vi "SID_test_dump_player.vi"() -> ()   [LabVIEW 2018]
doc: "This VI illustrates how to generate and play sine, square, sawtooth and triangle waveforms. You can change the frequency and type of the waveform generated as it plays continuously."
uses:
  SID_voice_reg.ctl
  SID_filter_reg.ctl
  <vilib>/sound2/lvsound2.llb/Sampling Mode.ctl
  <vilib>/sound2/lvsound2.llb/Sound Data Format.ctl
  <vilib>/sound2/lvsound2.llb/Sound Output Set Volume (Single).vi
  <vilib>/sound2/lvsound2.llb/Sound Output Write (DBL Single).vi
panel:
  in  "Filter":T1 {"vol" format="%0.2f"; "res" format="%0.2f"; "freq" format="%0.2f"}
  in  "VC3":T2 {"Duty" format="%0.2f"; "ADSR"."R" format="%0.2f"; "ADSR"."S" format="%0.2f"; "ADSR"."D" format="%0.2f"; "ADSR"."A" format="%0.2f"; "freq" format="%0.2f"}
  in  "VC1":T2 {"Duty" format="%0.2f"; "ADSR"."R" format="%0.2f"; "ADSR"."S" format="%0.2f"; "ADSR"."D" format="%0.2f"; "ADSR"."A" format="%0.2f"; "freq" format="%0.2f"}
  in  "VC2":T2 {"Duty" format="%0.2f"; "ADSR"."R" format="%0.2f"; "ADSR"."S" format="%0.2f"; "ADSR"."D" format="%0.2f"; "ADSR"."A" format="%0.2f"; "freq" format="%0.2f"}
  out "VC3":dbl[](graph)
  out "VC2":dbl[](graph)
  out "VC1":dbl[](graph)
  out "data size(s)":i32
  out "time Audio":u32
  out "time SID":u32
  in  "Volume":dbl=0.5
  out "Wave":dbl[](graph)
  in  "Stop":bool
  in  "Device ID":u32
  # "D:\\work\\experimets\\C64\\a_mind_is_born_LV.wav"
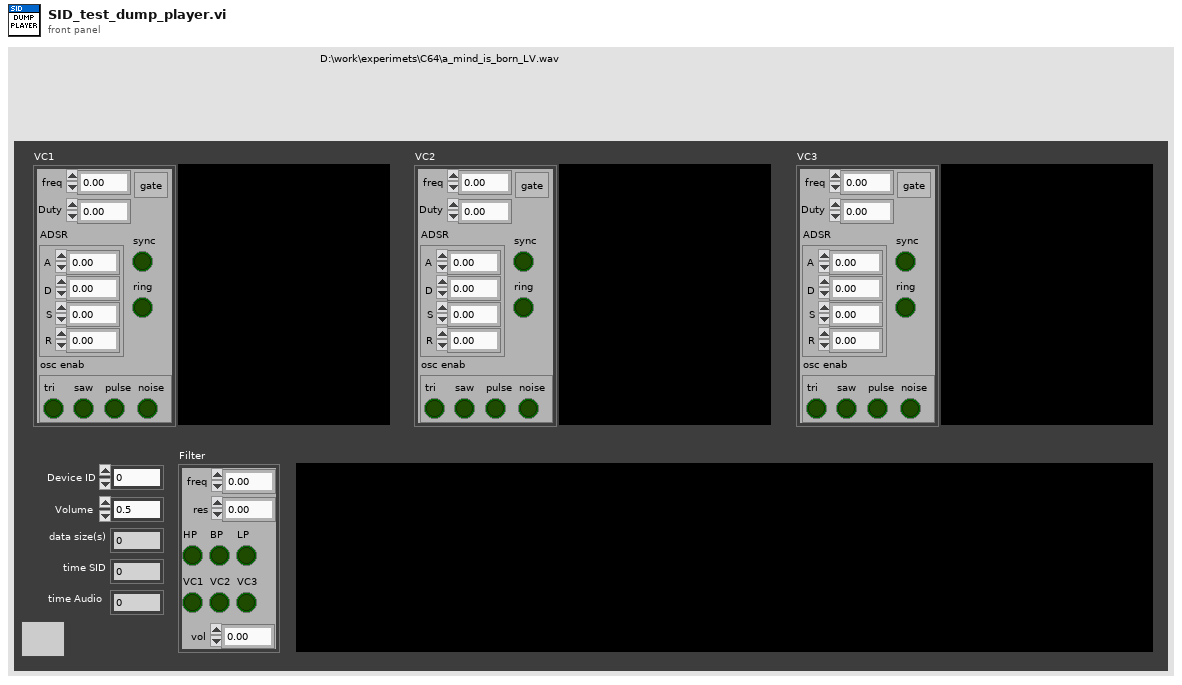
[diagram p1: front panel]
types:
  T1 = typedef "SID_filter_reg.ctl" = cluster{"freq":dbl, "res":dbl, "HP":bool, "BP":bool, "LP":bool, "VC1":bool, "VC2":bool, "VC3":bool, "vol":dbl}
  T2 = typedef "SID_voice_reg.ctl" = cluster{"freq":dbl, "gate":bool, "ADSR":cluster{"A":dbl, "D":dbl, "S":dbl, "R":dbl}, "Duty":dbl, "osc enab":cluster{"tri":bool, "saw":bool, "pulse":bool, "noise":bool}, "sync":bool, "ring":bool}
  T3 = enum16{"idle", "pre-attack", "attack", "pre-decay", "decay", "sustain", "pre-release", "release"}
  T4 = typedef "Sound Data Format.ctl" = cluster{"sample rate (S/s)":dbl, "number of channels":i32, "bits per sample":i32}
  T5 = typedef "Sampling Mode.ctl" = i32
  T6 = typedef "Sound Output Task ID.ctl" = u32
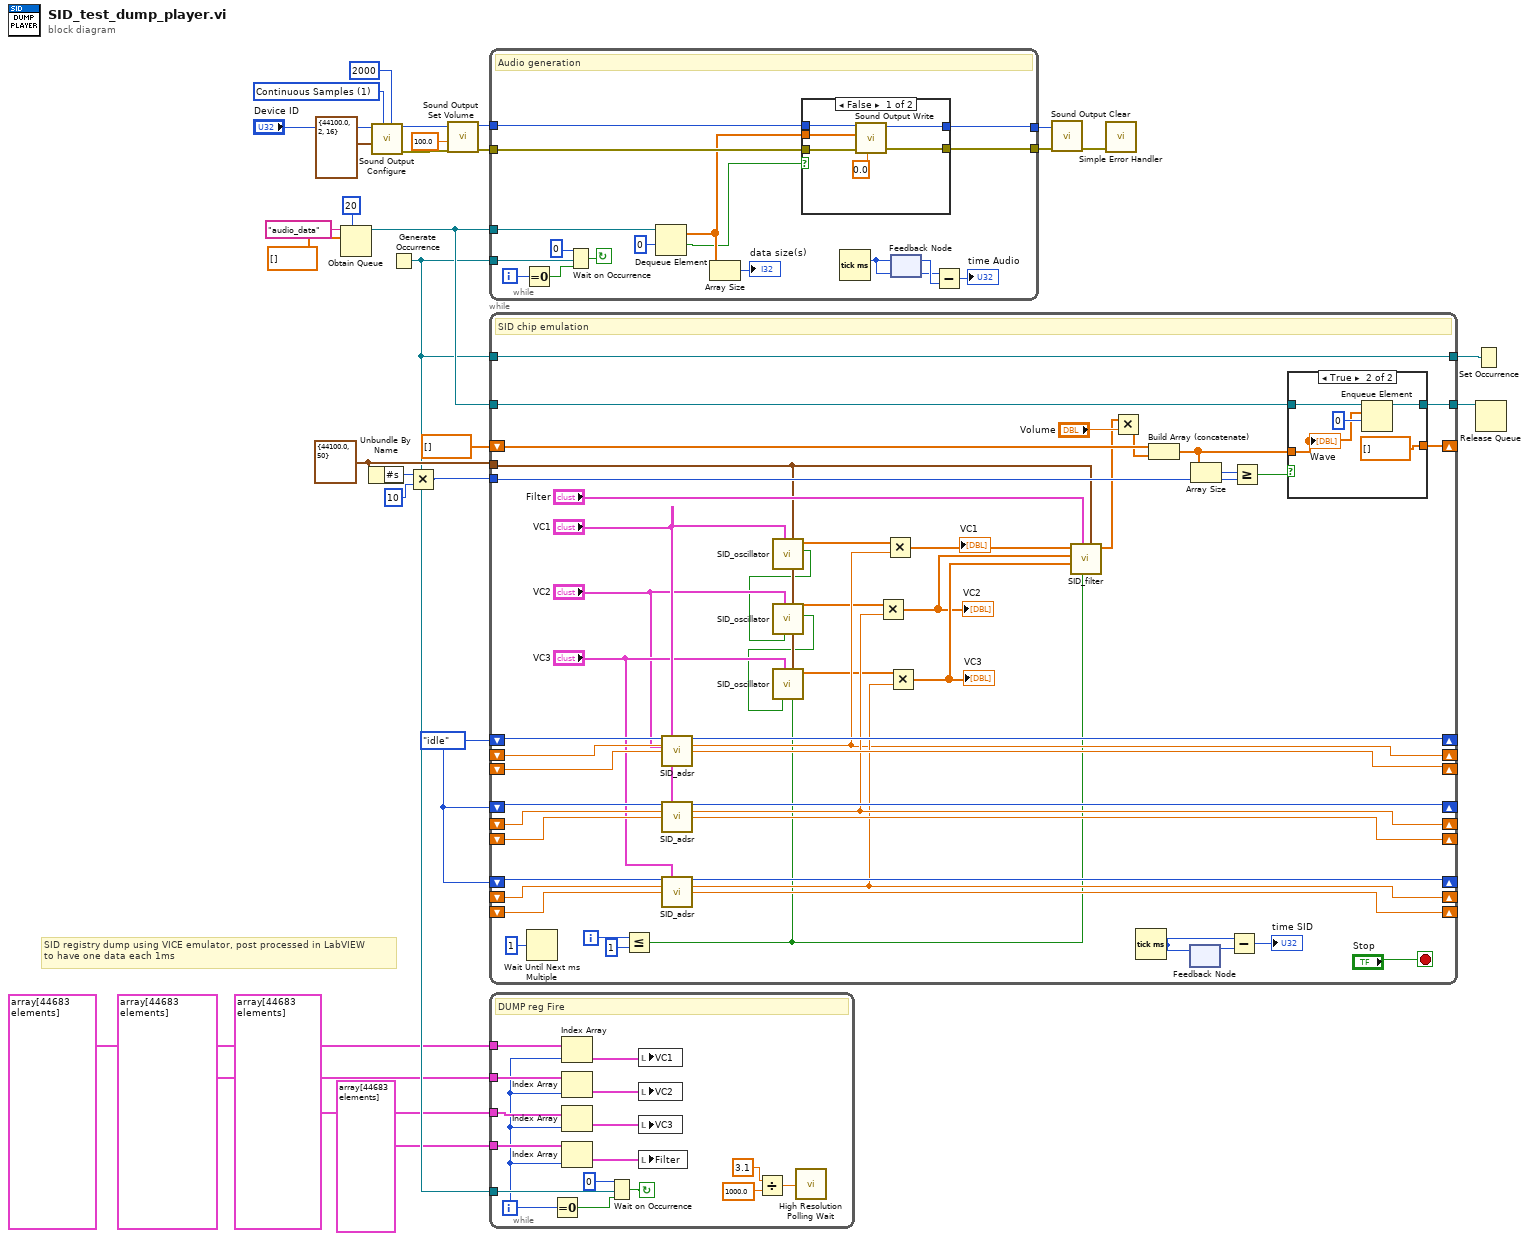
[diagram p0: block diagram]
diagram:
  w9 = cluster{"Fs":dbl, "#s":i32} {"Fs"=44100.0, "#s"=50} ("sampling info")
  w5 = T3."idle"
  w28 = T5 1 items=["Finite Samples", "Continuous Samples"] ("sample mode")
  # "SID registry dump using VICE emulator, post processed in LabVIEW\nto have one data each 1ms"
  n1 = Obtain Queue(max queue size (-1, unlimited)=20, name (unnamed)="audio_data", element data type=dbl[] []) -> (queue out=w16:refnum<queue>)  [unwired: 2 in, 2 out]
  n2 = Unbundle By Name(w9) -> ("#s"=w11:i32)
  n3 = call <vilib>:"Sound Output Configure.vi"("number of samples/ch"=2000 ("Number of Samples/ch"), "sample mode"=w28, "sound format"=T4 {"sample rate (S/s)"=44100.0, "number of channels"=2, "bits per sample"=16} ("Sound Format"), "device ID"="Device ID") -> ("error out"=w25:errorcluster, "task ID"=w23:T6)  [unwired: 6 in]
  n4 = Generate Occurrence() -> (w7:refnum<k4>)
  n5 = Multiply(x=w11, y=10) -> (x*y=w8:i32)
  n6 = call-poly <vilib>:"Sound Output Set Volume.vi"("error in (no error)"=w25, "volume"=100.0, "task ID"=w23) -> ("error out"=w21:errorcluster, "task ID out"=w22:T6)  [unwired: 7 in]
  n7 = while {
    tunnel: w22 -> [w38]
    tunnel: w21 -> [w39]
    tunnel: [w35] -> w20
    tunnel: [w34] -> w19
    tunnel: w7 -> [w46]
    tunnel: w16 -> [w36]
    i -> [w40]
    stop <- w44 continue-if-true
    # "Audio generation"
    n8 = Equal To 0?(x=w40) -> (x = 0?=w32:bool)
    n9 = Wait on Occurrence(1:w32, 2:w46, 3:0 ("ms timeout (-1)")) -> (0:w44:bool)
    n10 = Dequeue Element(queue=w36, timeout in ms (-1)=0) -> (element=w31:dbl[], timed out?=w30:bool)  [unwired: 1 in, 2 out]
    n11 = Array Size(array=w31) -> (size(s)=→"data size(s)":i32)
    n12 = case shown="False" w30 {
      tunnel: w39 -> [w52 w53]
      tunnel: w38 -> [w51 w54]
      tunnel: [w49 w54] -> w35
      tunnel: [w48 w53] -> w34
      tunnel: w31 -> [w47 _]
      frame False {
        n13 = call-poly <vilib>:"Sound Output Write.vi"("timeout (sec)"=0.0, "error in (no error)"=w52, "data"=w47, "task ID"=w51) -> ("error out"=w48:errorcluster, "task ID out"=w49:T6)  [unwired: 6 in]
      }
      frame True {
      }
    }
    n14 = Tick Count (ms)() -> (millisecond timer value=w41:u32)
    n15 = feedback #1() -> (w42:u32)  [unwired: 1 in]
    n16 = feedback-in #1(w41) -> ()
    n17 = Subtract(x=w41, y=w42) -> (x-y=→"time Audio":u32)
  }
  n18 = while {
    shift-right: [w88] -> _
    shift-left: _ -> [w89]
    shift-right: [w68] -> _
    shift-left: _ -> [w90]
    shift-right: [w87] -> _
    shift-left: w5 -> [w91]
    tunnel: w7 -> [w101]
    tunnel: [w101] -> w18
    tunnel: w16 -> [w98]
    tunnel: [w97] -> w15
    shift-right: [w92] -> _
    shift-left: dbl[] [] -> [w96]
    shift-right: [w82] -> _
    shift-left: _ -> [w83]
    shift-right: [w74] -> _
    shift-left: _ -> [w84]
    shift-right: [w81] -> _
    shift-left: w5 -> [w85]
    tunnel: w9 -> [w66]
    shift-right: [w79] -> _
    shift-left: _ -> [w78]
    shift-right: [w73] -> _
    shift-left: _ -> [w77]
    shift-right: [w80] -> _
    shift-left: w5 -> [w76]
    tunnel: w8 -> [w75]
    i -> [w65]
    stop <- "Stop" stop-if-true
    # "SID chip emulation"
    n19 = Wait Until Next ms Multiple(millisecond multiple=u32 1) -> ()  [unwired: 1 out]
    n20 = Less Or Equal?(x=w65, y=1) -> (x <= y?=w58:bool)
    n21 = call "SID_adsr.vi"("status in"=w91, "Reg"="VC1", "mod in"=w90, "acc in"=w89) -> ("status out"=w87:T3, "mod out"=w68:dbl, "acc out"=w88:dbl)  [unwired: 9 in]
    n22 = call "SID_adsr.vi"("status in"=w85, "Reg"="VC2", "mod in"=w84, "acc in"=w83) -> ("status out"=w81:T3, "mod out"=w74:dbl, "acc out"=w82:dbl)  [unwired: 9 in]
    n23 = call "SID_adsr.vi"("status in"=w76, "Reg"="VC3", "mod in"=w77, "acc in"=w78) -> ("status out"=w80:T3, "mod out"=w73:dbl, "acc out"=w79:dbl)  [unwired: 9 in]
    n24 = call "SID_oscillator.vi"("reset phase"=w58, "sampling info"=w66, "Reg"="VC1") -> ("MSB out"=w59:bool, "wave"=w57:dbl[])  [unwired: 7 in]
    n25 = call "SID_oscillator.vi"("reset phase"=w58, "sampling info"=w66, "MSB in"=w59, "Reg"="VC2") -> ("MSB out"=w55:bool, "wave"=w60:dbl[])  [unwired: 6 in]
    n26 = call "SID_oscillator.vi"("reset phase"=w58, "sampling info"=w66, "MSB in"=w55, "Reg"="VC3") -> ("wave"=w56:dbl[])  [unwired: 6 in, 1 out]
    n27 = Multiply(x=w60, y=w74) -> (x*y=w67:dbl[])
    "VC2" <- w67
    n28 = Multiply(x=w57, y=w68) -> (x*y=w71:dbl[])
    "VC1" <- w71
    n29 = Multiply(x=w56, y=w73) -> (x*y=w70:dbl[])
    "VC3" <- w70
    n30 = call "SID_filter.vi"("sampling info"=w66, "reset"=w58, "filter"="Filter", "VC3"=w70, "VC2"=w67, "VC1"=w71) -> ("out"=w72:dbl[])  [unwired: 5 in]
    n31 = Multiply(x=w72, y="Volume") -> (x*y=w86:dbl[])
    n32 = Tick Count (ms)() -> (millisecond timer value=w105:u32)
    n33 = Build Array (concatenate)(w96, w86) -> (w93:dbl[])
    n34 = feedback-in #2(w105) -> ()
    n35 = feedback #2() -> (w104:u32)  [unwired: 1 in]
    n36 = Array Size(array=w93) -> (size(s)=w95:i32)
    n37 = Subtract(x=w105, y=w104) -> (x-y=→"time SID":u32)
    n38 = Greater Or Equal?(x=w95, y=w75) -> (x >= y?=w94:bool)
    n39 = case shown="True" w94 {
      tunnel: w98 -> [w106 w112]
      tunnel: [w106 w111] -> w97
      tunnel: w93 -> [w107 w108]
      tunnel: [w107 dbl[] []] -> w92
      frame False {
      }
      frame True {
        n40 = Enqueue Element(queue=w112, element=w108, timeout in ms (-1)=0) -> (queue out=w111:refnum<queue>)  [unwired: 1 in, 2 out]
        "Wave" <- w108
      }
    }
  }
  n41 = while {
    tunnel: w7 -> [w126]
    tunnel: T1[] array[44683 elements] ("filter") -> [w124]
    tunnel: T2[] array[44683 elements] ("Array") -> [w123]
    tunnel: T2[] array[44683 elements] ("voice 2") -> [w122]
    tunnel: T2[] array[44683 elements] ("voice 1") -> [w125]
    i -> [w121]
    stop <- w120 continue-if-true
    # "DUMP reg Fire"
    n42 = Equal To 0?(x=w121) -> (x = 0?=w127:bool)
    n43 = Index Array(array=w125, index=w121) -> (element=w119:T2)
    n44 = Index Array(array=w122, index=w121) -> (element=w118:T2)
    n45 = Index Array(array=w123, index=w121) -> (element=w113:T2)
    n46 = Index Array(array=w124, index=w121) -> (element=w117:T1)
    n47 = Wait on Occurrence(1:w127, 2:w126, 3:0 ("ms timeout (-1)")) -> (0:w120:bool)
    n48 = local write "VC1"(w119) -> ()
    n49 = local write "VC2"(w118) -> ()
    n50 = local write "VC3"(w113) -> ()
    n51 = local write "Filter"(w117) -> ()
    n52 = Divide(x=3.1 ("mseconds to wait"), y=1000.0) -> (x/y=w115:dbl)
    n53 = call <vilib>:"High Resolution Polling Wait.vi"("seconds to wait"=w115) -> ()  [unwired: 10 in, 1 out]
  }
  n54 = call <vilib>:"Sound Output Clear.vi"("error in (no error)"=w19, "task ID"=w20) -> ("error out"=w26:errorcluster)  [unwired: 9 in]
  n55 = call <vilib>:"Simple Error Handler.vi"("error in (no error)"=w26) -> ()  [unwired: 4 in, 5 out]
  n56 = Set Occurrence(w18) -> ()
  n57 = Release Queue(queue=w15) -> ()  [unwired: 2 in, 3 out]
